vi "TestHelper_GUID.vi"() -> (3 "GUID":string)   [LabVIEW 2017]
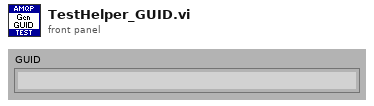
[diagram p1: front panel]
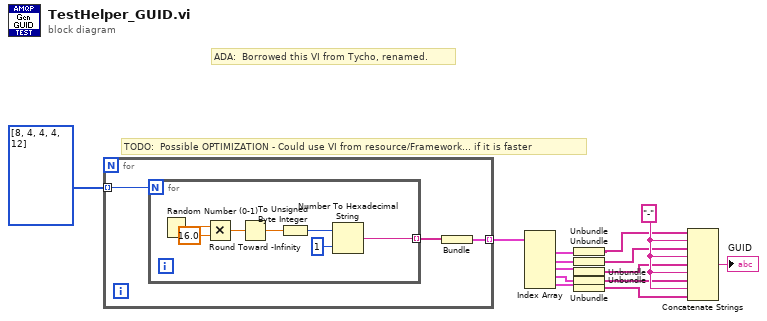
[diagram p0: block diagram]
diagram:
  w12 = "-"
  # "ADA:  Borrowed this VI from Tycho, renamed."
  # "TODO:  Possible OPTIMIZATION - Could use VI from resource/Framework... if it is faster"
  n1 = for {
    tunnel: i32[] [8, 4, 4, 4, 12] -> [w16] mode=indexing
    tunnel: [w15] -> w13 mode=indexing
    n2 = for {
      N: w16 -> [_]
      tunnel: [w18] -> w17 mode=indexing
      n3 = Random Number (0-1)() -> (number: 0 to 1=w24:dbl)
      n4 = Multiply(x=w24, y=16.0) -> (x*y=w22:dbl)
      n5 = Round Toward -Infinity(1:w22) -> (0:w21:dbl)
      n6 = To Unsigned Byte Integer(number=w21) -> (unsigned 8bit integer=w20:u8)
      n7 = Number To Hexadecimal String(1:i16 1 ("width (-)"), 2:w20) -> (0:w18:string)
    }
    n8 = Bundle(w17) -> (w15:cluster{string[]})  [unwired: 1 in]
  }
  n9 = Index Array(array=w13) -> (element #1=w11:cluster{string[]}, element #2=w10:cluster{string[]}, element #3=w9:cluster{string[]}, element #4=w8:cluster{string[]}, element #5=w7:cluster{string[]})  [unwired: 5 in]
  n10 = Unbundle(w11) -> (w6:string[])
  n11 = Unbundle(w10) -> (w5:string[])
  n12 = Unbundle(w9) -> (w4:string[])
  n13 = Unbundle(w8) -> (w3:string[])
  n14 = Unbundle(w7) -> (w2:string[])
  n15 = Concatenate Strings(w6, w12, w5, w12, w4, w12, w3, w12, w2) -> (→"GUID":string)
